vi "Init Events.vi"(8 "error in (no error)":errorcluster, 11 "InfoService in":refnum<class "NodeStatus.lvclass">) -> (0 "error out":errorcluster, 3 "InfoService out":refnum<class "NodeStatus.lvclass">)   [LabVIEW 2020, in "Vecto.lvlib" / "NodeStatus.lvclass"]
uses:
  NodeStatus.lvclass
  lv-promises/Promises/Promise/Promise.lvclass
  Incoming Events.ctl
  Task Status Data.ctl
  Node Info Data.ctl
  Node Info.ctl
  Task Info.ctl
  NodeStatus.lvclass/NodeStatus.ctl
  VectoConfig/VectoConfig.lvlib
  Vecto.lvlib
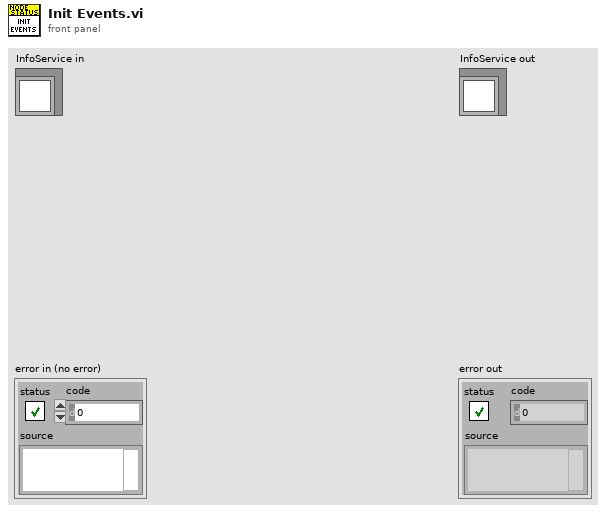
[diagram p1: front panel]
types:
  T1 = typedef "Vecto.lvlib/NodeStatus.lvclass/Node Info Data.ctl" = cluster{"Node Info":T2}
  T2 = typedef "Vecto.lvlib/Node Info.ctl" = cluster{"Name":string, "ID":u32, "Status":string, "SWVersion":string, "ConfigVersion":string, "Tasks":T3[]}
  T3 = typedef "VectoConfig.lvlib/Task Info.ctl" = cluster{"Name":string, "Status":string}
  T4 = typedef "Vecto.lvlib/NodeStatus.lvclass/Task Status Data.ctl" = cluster{"Name":string, "Status":string}
  T5 = typedef "Vecto.lvlib/NodeStatus.lvclass/Incoming Events.ctl" = cluster{"Info Request":refnum<user-event>, "Update Task":refnum<user-event>, "Update Info":refnum<user-event>, "Close":refnum<user-event>}
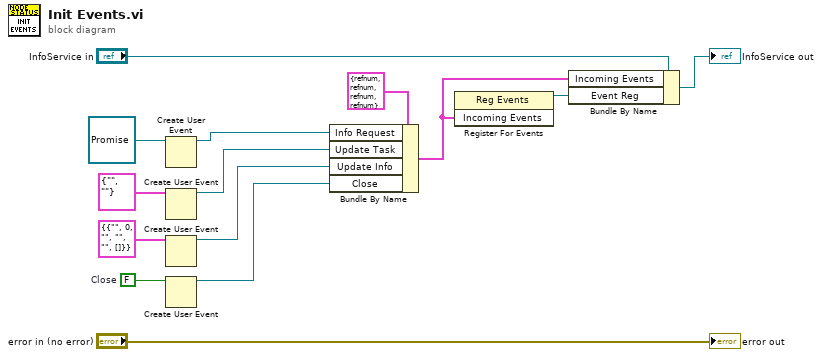
[diagram p0: block diagram]
diagram:
  w2 = FALSE  # Close
  n1 = Create User Event(user event datatype=refnum<class "Promise.lvclass"> refnum ("Futures:Promise")) -> (user event=w12:refnum<user-event>)  [unwired: 1 in, 1 out]
  n2 = Create User Event(user event datatype=T4 {"Name"="", "Status"=""} ("Task Status Data")) -> (user event=w5:refnum<user-event>)  [unwired: 1 in, 1 out]
  n3 = Create User Event(user event datatype=T1 {"Node Info"={"Name"="", "ID"=0, "Status"="", "SWVersion"="", "ConfigVersion"="", "Tasks"=[]}} ("Node Info Data")) -> (user event=w3:refnum<user-event>)  [unwired: 1 in, 1 out]
  n4 = Create User Event(user event datatype=w2) -> (user event=w1:refnum<user-event>)  [unwired: 1 in, 1 out]
  n5 = Bundle By Name(cluster=T5 {"Info Request"=refnum, "Update Task"=refnum, "Update Info"=refnum, "Close"=refnum} ("Incoming Events"), "Info Request"=w12, "Update Task"=w5, "Update Info"=w3, "Close"=w1) -> (w10:T5)
  n6 = register-events(w10) -> (reference out=w9:refnum<event-registration>)  [unwired: 2 in, 1 out]
  n7 = Bundle By Name(cluster="InfoService in", "Incoming Events"=w10, "Event Reg"=w9) -> (→"InfoService out":refnum<class "NodeStatus.lvclass">)
  "error out" <- "error in (no error)"
